vi "运行调试UI.vi"() -> ()   [LabVIEW 2016, in "EXO2-Sonde.lvlib"]
uses:
  EXO2-Sonde.lvlib
  <vilib>/Utility/miscctls.llb/LVPointTypeDef.ctl
  Var/Holding Var.vi
  Var/Input Var.vi
  <vilib>/ptbypt/NI_PtbyPt.lvlib
panel:
  in  "测试间隔（H）":u16=1
  in  "EXO启用":bool
  in  "baud rate (9600)":u32=38400
  in  "EXO串口":refnum<visa-resource-name>="COM4"
  out "EXO原始数据包":string
  in  "停止":bool
  in  "启动":bool
  out "EXO message":T1
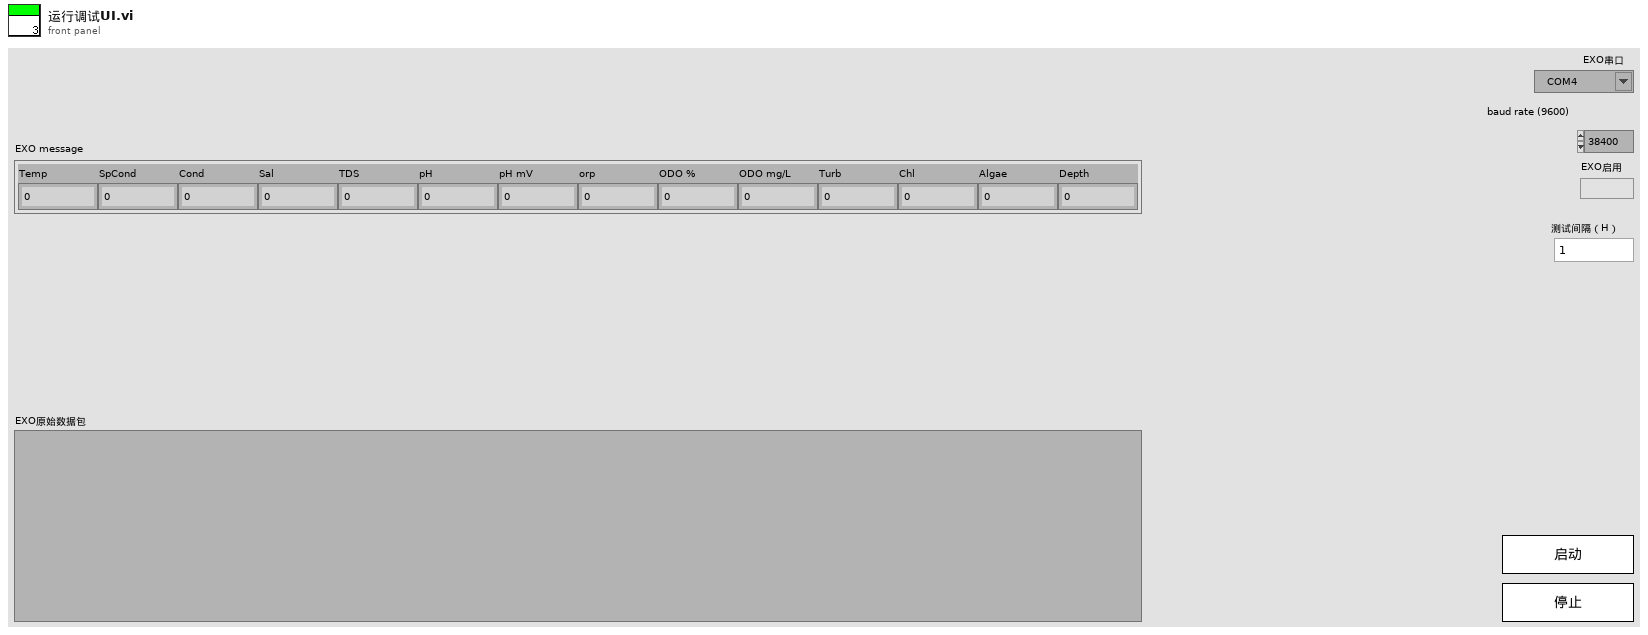
[diagram p1: front panel]
types:
  T1 = cluster{"Temp":dbl, "SpCond":dbl, "Cond":dbl, "Sal":dbl, "TDS":dbl, "pH":dbl, "pH mV":dbl, "orp":dbl, "ODO %":dbl, "ODO mg/L":dbl, "Turb":dbl, "Chl":dbl, "Algae":dbl, "Depth":dbl}
  T2 = typedef "LVPointTypeDef.ctl" = cluster{"Horizontal":i16, "Vertical":i16}
  T3 = enum8{"Enabled", "Disabled", "Disabled and Grayed Out"}
  T4 = typedef "LVDateTimeRec.ctl" = cluster{"秒数的小数部分":dbl, "秒":i32, "分":i32, "时":i32, "日":i32, "月":i32, "年":i32, "天数（周）":i32, "天数（年）":i32, "DST":i32}
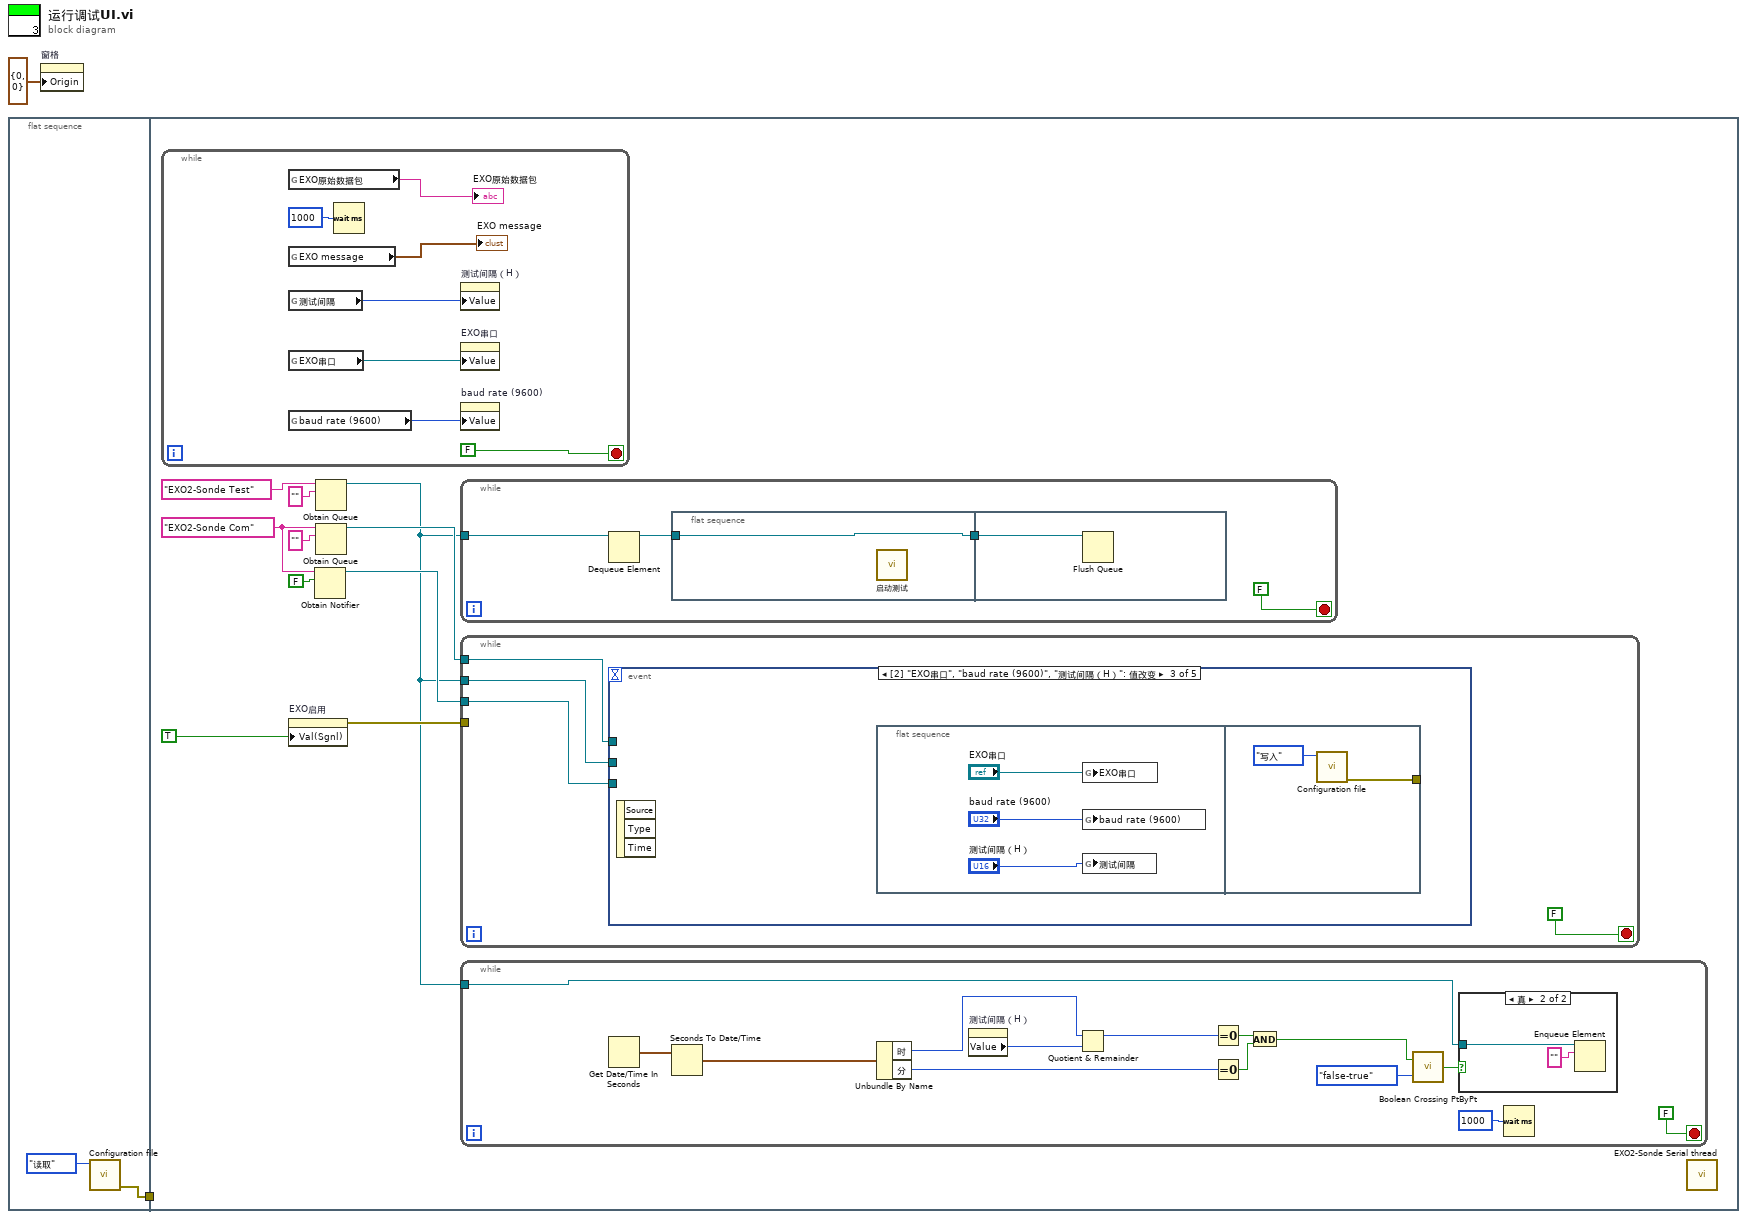
[diagram p0: block diagram]
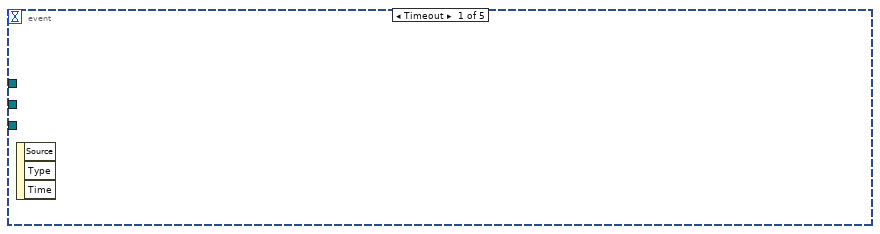
[diagram p3: hidden frame]
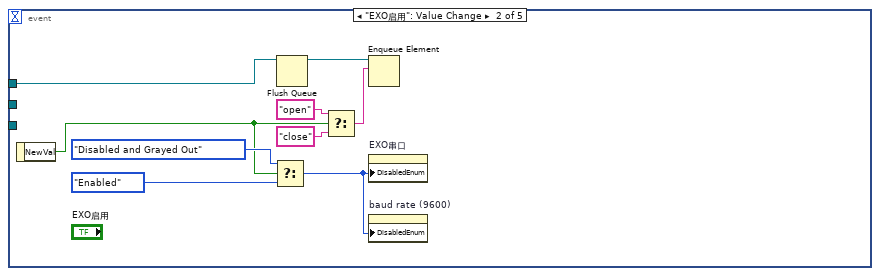
[diagram p4: hidden frame]
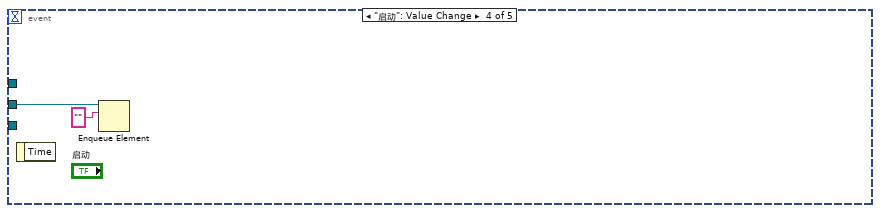
[diagram p5: hidden frame]
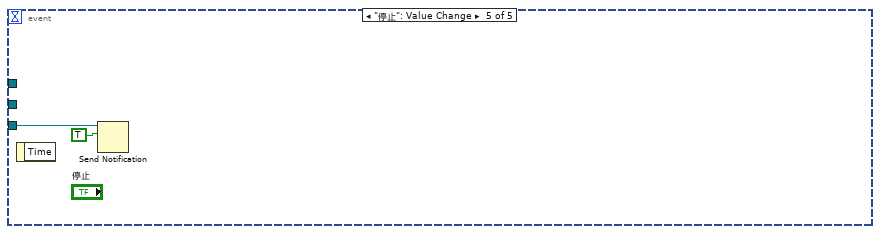
[diagram p6: hidden frame]
diagram:
  n1 = flat-sequence {
    tunnel: [w3] -> w1
    tunnel: w1 -> [_]
    frame #0 {
      n2 = call "Configuration file.vi"("类型"=enum16{"读取", "写入"}."读取") -> ("error out"=w3:errorcluster)  [unwired: 10 in]
    }
    frame #1 {
      w13 = "EXO2-Sonde Com" ("名称（未命名）")
      n3 = while {
        stop <- FALSE stop-if-true
        n4 = global read "Input Var.vi" "EXO原始数据包"() -> (→"EXO原始数据包":string)
        n5 = global read "Input Var.vi" "EXO message"() -> (→"EXO message":T1)
        n6 = global read "Holding Var.vi" "测试间隔"() -> (w37:u16)
        n7 = global read "Holding Var.vi" "EXO串口"() -> (w40:refnum<visa-resource-name>)
        n8 = global read "Holding Var.vi" "baud rate (9600)"() -> (w39:u32)
        n9 = Wait (ms)(milliseconds to wait=u32 1000 ("等待时间（毫秒）")) -> ()  [unwired: 1 out]
        n10 = property on="测试间隔（H）" class="DigNum (严格)"("Value"=w37) -> ()  [unwired: 2 in, 2 out]
        n11 = property on="EXO串口" class="VISAName"("Value"=w40) -> ()  [unwired: 2 in, 2 out]
        n12 = property on="baud rate (9600)" class="DigNum (严格)"("Value"=w39) -> ()  [unwired: 2 in, 2 out]
      }
      n13 = property on="EXO启用" class="Bool (严格)"("Val(Sgnl)"=TRUE ("EXO启用")) -> (error out=w7:errorcluster)  [unwired: 2 in, 1 out]
      n14 = Obtain Notifier(name (unnamed)=w13, notification data type=FALSE) -> (notifier out=w10:refnum<notifier>)  [unwired: 2 in, 2 out]
      n15 = Obtain Queue(name (unnamed)="EXO2-Sonde Test" ("名称（未命名）"), element data type="") -> (queue out=w5:refnum<queue>)  [unwired: 3 in, 2 out]
      n16 = Obtain Queue(name (unnamed)=w13, element data type="") -> (queue out=w11:refnum<queue>)  [unwired: 3 in, 2 out]
      n17 = while {
        tunnel: w5 -> [w34]
        stop <- FALSE stop-if-true
        n18 = Dequeue Element(queue=w34) -> (queue out=w33:refnum<queue>)  [unwired: 2 in, 3 out]
        n19 = flat-sequence {
          tunnel: w33 -> [w35]
          tunnel: [w35] -> w32
          tunnel: w32 -> [w36]
          frame #0 {
            n20 = call "启动测试.vi"() -> ()  [unwired: 12 in]
          }
          frame #1 {
            n21 = Flush Queue(queue=w36) -> ()  [unwired: 1 in, 3 out]
          }
        }
      }
      n22 = while {
        tunnel: w11 -> [w46]
        tunnel: w10 -> [w45]
        tunnel: w5 -> [w44]
        tunnel: w7 -> [_]
        stop <- FALSE stop-if-true
        n23 = event shown="[2] \"EXO串口\", \"baud rate (9600)\", \"测试间隔（H）\": 值改变" {
          selector: _ -> [_ _ _ _ _]
          dyn-events: _ -> [_ _ _ _ _]
          timeout: _ -> [_ _ _ _ _]
          tunnel: w46 -> [_ w49 _ _ _]
          tunnel: w45 -> [_ _ _ _ w65]
          tunnel: w44 -> [_ _ _ w63 _]
          event Timeout {
            n24 = event-data() -> ()  [unwired: 1 in, 3 out]
          }
          event "EXO启用": Value Change {
            n25 = event-data() -> ("NewVal"=w48:bool)  [unwired: 1 in]
            n26 = Select(t=T3."Disabled and Grayed Out" ("禁用"), s=w48, f=T3."Enabled" ("禁用")) -> (s? t:f=w54:T3)
            n27 = Flush Queue(queue=w49) -> (queue out=w51:refnum<queue>)  [unwired: 1 in, 2 out]
            n28 = Select(t="open", s=w48, f="close") -> (s? t:f=w50:string)
            n29 = Enqueue Element(queue=w51, element=w50) -> ()  [unwired: 2 in, 3 out]
            n30 = property on="EXO串口" class="VISAName"("DisabledEnum"=w54) -> ()  [unwired: 2 in, 2 out]
            n31 = property on="baud rate (9600)" class="DigNum (严格)"("DisabledEnum"=w54) -> ()  [unwired: 2 in, 2 out]
          }
          event "EXO串口", "baud rate (9600)", "测试间隔（H）": Value Change {
            n32 = event-data() -> ()  [unwired: 1 in, 3 out]
            n33 = flat-sequence {
              tunnel: [w60] -> _
              frame #0 {
                n34 = global write "Holding Var.vi" "EXO串口"("EXO串口") -> ()
                n35 = global write "Holding Var.vi" "baud rate (9600)"("baud rate (9600)") -> ()
                n36 = global write "Holding Var.vi" "测试间隔"("测试间隔（H）") -> ()
              }
              frame #1 {
                n37 = call "Configuration file.vi"("类型"=enum16{"读取", "写入"}."写入") -> ("error out"=w60:errorcluster)  [unwired: 10 in]
              }
            }
          }
          event "启动": Value Change {
            n38 = event-data() -> ()  [unwired: 1 in, 1 out]
            n39 = Enqueue Element(queue=w63, element="" ("元素")) -> ()  [unwired: 2 in, 3 out]
          }
          event "停止": Value Change {
            n40 = event-data() -> ()  [unwired: 1 in, 1 out]
            n41 = Send Notification(notification=TRUE ("通知"), notifier=w65) -> ()  [unwired: 1 in, 2 out]
          }
        }
      }
      n42 = while {
        tunnel: w5 -> [w16]
        stop <- FALSE stop-if-true
        n43 = Get Date/Time In Seconds() -> (seconds since 1Jan1904=w26:timestamp)
        n44 = Seconds To Date/Time(time stamp (now)=w26) -> (date time rec=w25:T4)  [unwired: 1 in]
        n45 = Unbundle By Name(w25) -> ("时"=w24:i32, "分"=w21:i32)
        n46 = property on="测试间隔（H）" class="DigNum (严格)"() -> ("Value"=w23:u16)  [unwired: 2 in, 2 out]
        n47 = Quotient & Remainder(x=w24, y=w23) -> (x-y*floor(x/y)=w22:i32)  [unwired: 1 out]
        n48 = Equal To 0?(x=w22) -> (x = 0?=w19:bool)
        n49 = Equal To 0?(x=w21) -> (x = 0?=w20:bool)
        n50 = And(x=w19, y=w20) -> (x .and. y?=w18:bool)
        n51 = call <vilib>:"Boolean Crossing PtByPt.vi"("direction"=enum16{"either", "false-true", "true-false"}."false-true", "input"=w18) -> ("crossing"=w15:bool)  [unwired: 1 in]
        n52 = case shown="真" w15 {
          tunnel: w16 -> [_ w30]
          frame False {
          }
          frame True {
            n53 = Enqueue Element(queue=w30, element="" ("元素")) -> ()  [unwired: 2 in, 3 out]
          }
        }
        n54 = Wait (ms)(milliseconds to wait=u32 1000 ("等待时间（毫秒）")) -> ()  [unwired: 1 out]
      }
      n55 = call "EXO2-Sonde Serial thread.vi"() -> ()  [unwired: 12 in]
    }
  }
  n56 = property on="窗格" class="Pane"("Origin"=T2 {"Horizontal"=0, "Vertical"=0} ("原点")) -> ()  [unwired: 2 in, 2 out]
